vi "TCP_connect.vi"(8 "error in (no error)":errorcluster, 10 "port":u16=9000, 11 "TCP_IP.lvclass (in)":refnum<class "TCP_IP.lvclass">) -> (0 "error out":errorcluster)   [LabVIEW 2013, in "TCP_IP.lvclass"]
uses:
  TCP_IP.lvclass
  Experiment/Globals.vi
  Experiment/Experiment.lvclass
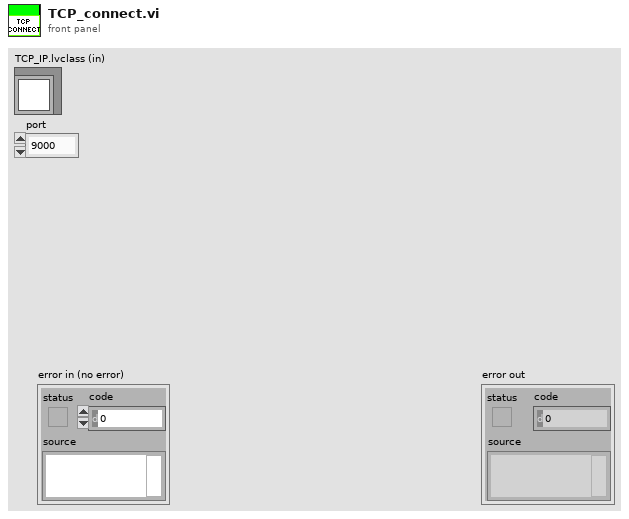
[diagram p1: front panel]
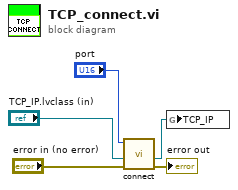
[diagram p0: block diagram]
diagram:
  n1 = call "connect.vi"("error in (no error)"="error in (no error)", "TCP_IP.lvclass (in)"="TCP_IP.lvclass (in)", "port"="port") -> ("error out"=→"error out":errorcluster, "TCP_IP.lvclass"=w1:refnum<class "TCP_IP.lvclass">)  [unwired: 7 in]
  n2 = global write "Globals.vi" "TCP_IP"(w1) -> ()
